vi "Set Node Text Content.vi"(8 "error in (no error)":errorcluster, 10 "node text":string, 11 "node in":refnum<k20>) -> (0 "error out":errorcluster, 3 "node out":refnum<k20>)   [LabVIEW 2014]
doc: "Returns the combined values of <B>Text_Node</B> children that the <B>node in</B> node owns."
uses:
  <vilib>/xml/Close Reference(Node).vi
  <vilib>/xml/NI_XML.lvlib
  <resource>/objmgr/DOMUserDefRef.rc
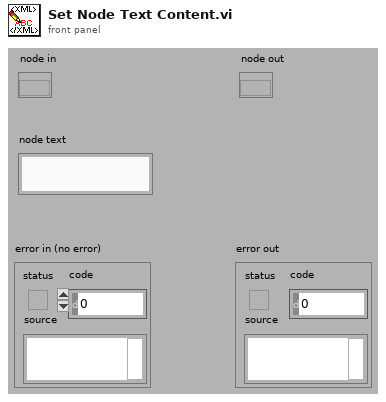
[diagram p1: front panel]
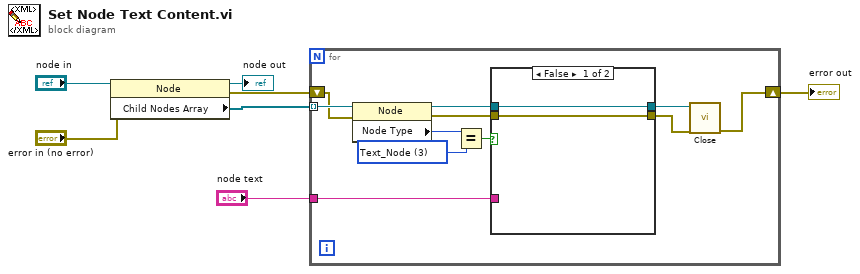
[diagram p0: block diagram]
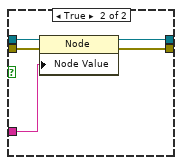
[diagram p2: hidden frame]
diagram:
  n1 = property class="Node"(reference="node in", error in="error in (no error)") -> (reference out=→"node out":refnum<k20>, error out=w5:errorcluster, "Child Nodes Array"=w4:refnum<k20>[])
  n2 = for {
    shift-right: [w9] -> w2
    shift-left: w5 -> [w17]
    tunnel: w4 -> [w18] mode=indexing
    tunnel: "node text" -> [w8]
    w15 = 3 items=["Element_Node"=1, "Attribute_Node"=2, "Text_Node"=3, "CDATASection_Node"=4, "EntityReference_Node"=5, "Entity_Node"=6, "ProcessingInstruction_Node"=7, "Comment_Node"=8, "Document_Node"=9, "DocumentType_Node"=10, "DocumentFragment_Node"=11, "Notation_Node"=12] ("Node Type")
    n3 = property class="Node"(reference=w18, error in=w17) -> (reference out=w13:refnum<k20>, error out=w12:errorcluster, "Node Type"=w16:i32)
    n4 = Equal?(x=w16, y=w15) -> (x = y?=w14:bool)
    n5 = case shown="False" w14 {
      tunnel: w13 -> [w20 w25]
      tunnel: w12 -> [w19 w24]
      tunnel: [w20 w23] -> w11
      tunnel: [w19 w22] -> w10
      tunnel: w8 -> [_ w21]
      frame False {
      }
      frame True {
        n6 = property class="Node"(reference=w25, error in=w24, "Node Value"=w21) -> (reference out=w23:refnum<k20>, error out=w22:errorcluster)
      }
    }
    n7 = call-poly <vilib>:"Close.vi"("error in (no error)"=w10, "node"=w11) -> ("error out"=w9:errorcluster)  [unwired: 7 out]
  }
  "error out" <- w2
